vi "dust_info.vi"(6 "timeout (25000ms)":i32=25000, 8 "error in (no error)":errorcluster, 11 "daemon reference in":refnum<k5>) -> (0 "error out":errorcluster, 1 "Cluster":T1, 2 "response":string, 3 "daemon reference out":refnum<k5>, 5 "command out":string="random")   [LabVIEW 2017]
doc: "<b>Command: </b>\"dust_info\"\n\n<b>Description: </b> This command request dust info from address dd.\n\n<b>Parameters: </b> None\n____________________________________________\nDIPC 692 Daemon API 10.0.0.1\nSam Tee - Dyson Technology Ltd\nCopyright (c) 2024, Dyson Technology Ltd"
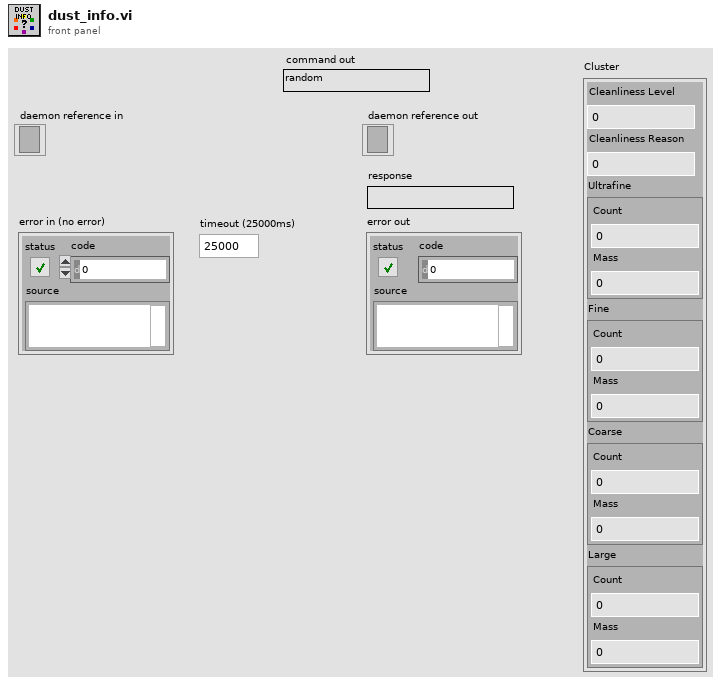
[diagram p1: front panel]
types:
  T1 = cluster{"Cleanliness Level":u32, "Cleanliness Reason":u32, "Ultrafine":cluster{"Count ":u32, "Mass":u32}, "Fine":cluster{"Count ":u32, "Mass":u32}, "Coarse":cluster{"Count ":u32, "Mass":u32}, "Large":cluster{"Count ":u32, "Mass":u32}}
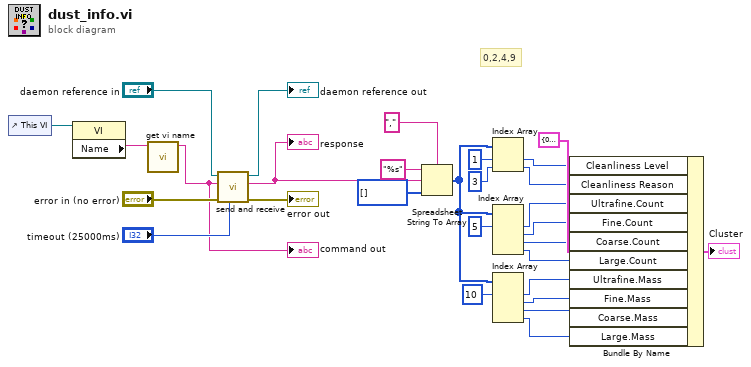
[diagram p0: block diagram]
diagram:
  # "0,2,4,9"
  n1 = control-ref of="This VI"() -> (w24:refnum<vi>)
  n2 = property class="VI"(reference=w24) -> ("Name"=w23:string)  [unwired: 1 in, 2 out]
  n3 = call "get vi name.vi"("library.lvlib:name.vi"=w23) -> ("vi name"=w22:string)  [unwired: 10 in]
  "command out" <- w22
  n4 = call "send and receive.vi"("timeout (25000ms)"="timeout (25000ms)", "error in (no error)"="error in (no error)", "command"=w22, "daemon reference in"="daemon reference in") -> ("error out"=→"error out":errorcluster, "response"=w19:string, "daemon reference out"=→"daemon reference out":refnum<k5>)  [unwired: 5 in]
  "response" <- w19
  n5 = Spreadsheet String To Array(delimiter (Tab)=",", format string="%s", spreadsheet string=w19, array type (2D Dbl)=u32[] []) -> (array=w6:u32[])
  n6 = Index Array(array=w6, index #1=1 ("index"), index #2=3 ("index")) -> (element #1=w13:u32, element #2=w12:u32)
  n7 = Index Array(array=w6, index #1=5 ("index")) -> (element #1=w10:u32, element #2=w9:u32, element #3=w8:u32, element #4=w7:u32)  [unwired: 3 in]
  n8 = Index Array(array=w6, index #1=10 ("index")) -> (element #1=w4:u32, element #2=w3:u32, element #3=w2:u32, element #4=w1:u32)  [unwired: 3 in]
  n9 = Bundle By Name(cluster=T1 {"Cleanliness Level"=0, "Cleanliness Reason"=0, "Ultrafine"={"Count "=0, "Mass"=0}, "Fine"={"Count "=0, "Mass"=0}, "Coarse"={"Count "=0, "Mass"=0}, "Large"={"Count "=0, "Mass"=0}} ("Cluster"), "Cleanliness Level"=w13, "Cleanliness Reason"=w12, "Ultrafine.Count"=w10, "Fine.Count"=w9, "Coarse.Count"=w8, "Large.Count"=w7, "Ultrafine.Mass"=w4, "Fine.Mass"=w3, "Coarse.Mass"=w2, "Large.Mass"=w1) -> (→"Cluster":T1)
